vi "tm_getparameterlimits_41.vi"(7 "Reconfigure (F)":bool, 8 "error in (no error)":errorcluster, 10 "Parameter":u32(ring)=4215968 items=["SENSOR MODE"=4212128, "SENSOR MODE LINE BUNDLE HEIGHT"=4212192, "READOUT DIRECTION"=4211904, "BIT PER CHANNEL"=4342976, "EXPOSURE TIME"=2049184, "CONTRAST GAIN"=3163312, "BINNING"=4215968, "TIMING READOUT TIME"=4223904, "INTERNAL FRAME RATE"=4225952, "INTERNAL FRAME INTERVAL"=4225968, "INTERNAL LINE SPEED"=4226000, "IMAGE WIDTH"=4343200, "IMAGE HEIGHT"=4343216, "IMAGE ROWBYTES"=4343232, "IMAGE FRAMEBYTES"=4343248, "IMAGE PIXEL TYPE"=4343296], 11 "Handle in":u32) -> (0 "error out":errorcluster, 2 "Limits":T1, 3 "Handle out":u32)   [LabVIEW 2023]
uses:
  tmcamcon.dll
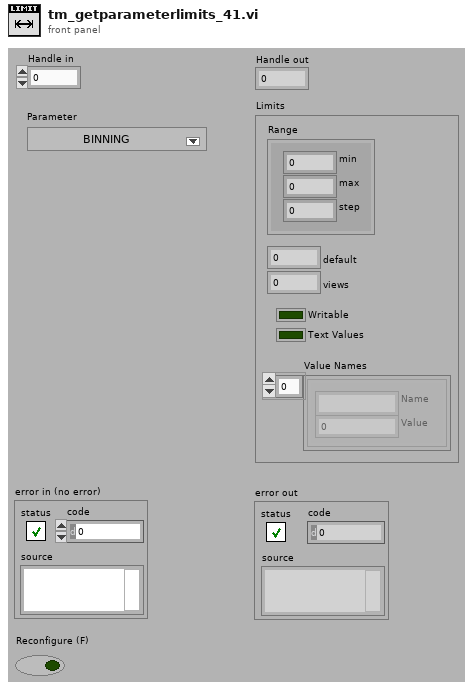
[diagram p1: front panel]
types:
  T1 = cluster{"Range":cluster{"min":dbl, "max":dbl, "step":dbl}, "default":dbl, "views":u32, "Writable":bool, "Text Values":bool, "Value Names":cluster{"Name":string, "Value":dbl}[]}
  T2 = cluster{"Property Name":string, "Property ID":i32}[]
  T3 = cluster{"Property Name":string, "Property ID":i32}
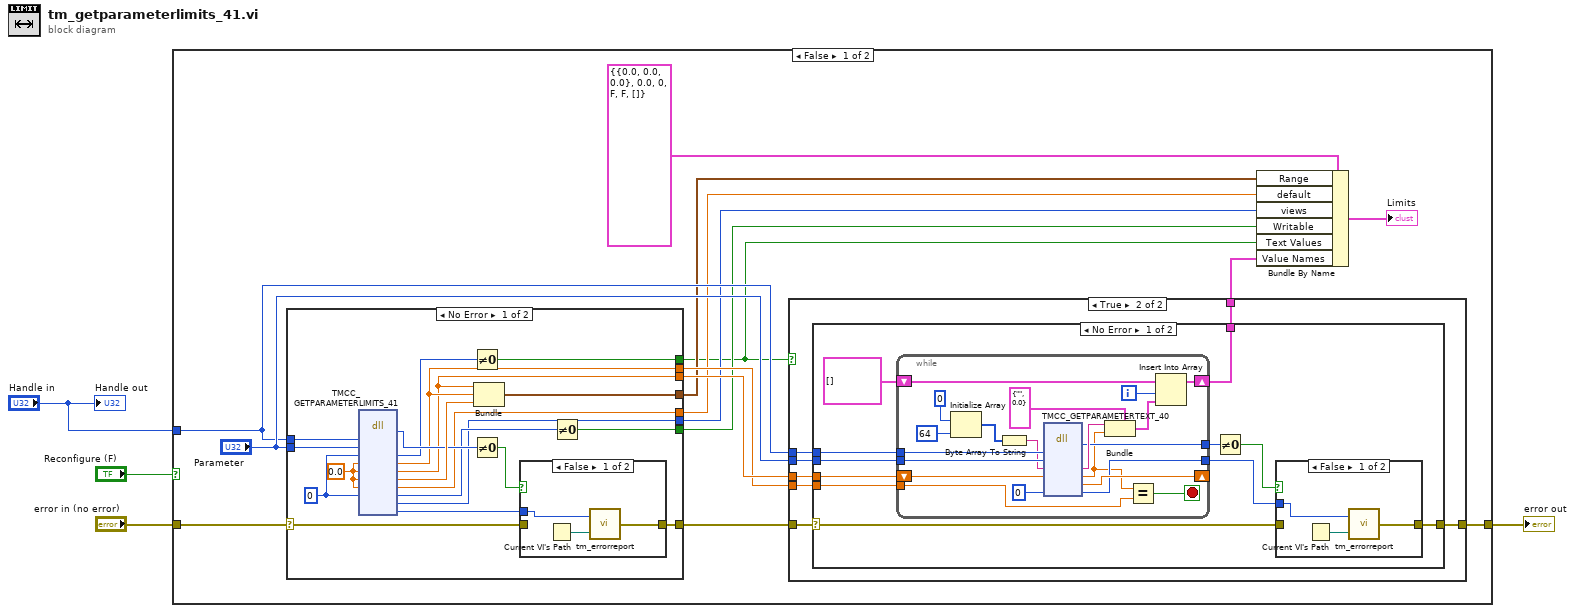
[diagram p0: block diagram]
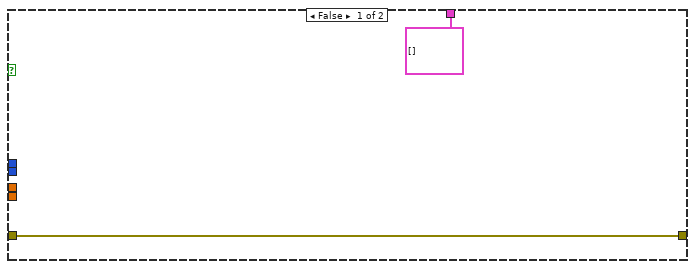
[diagram p2: hidden frame]
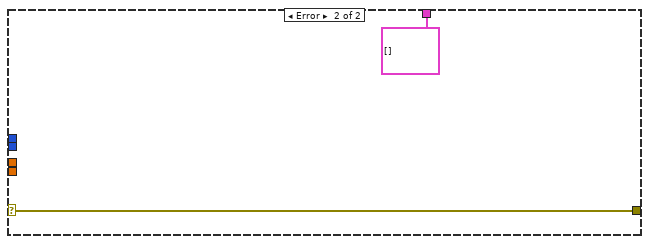
[diagram p4: hidden frame]
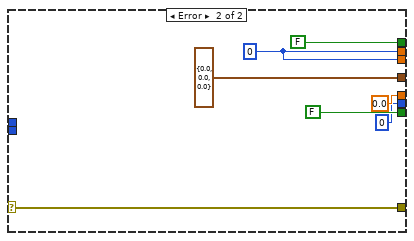
[diagram p6: hidden frame]
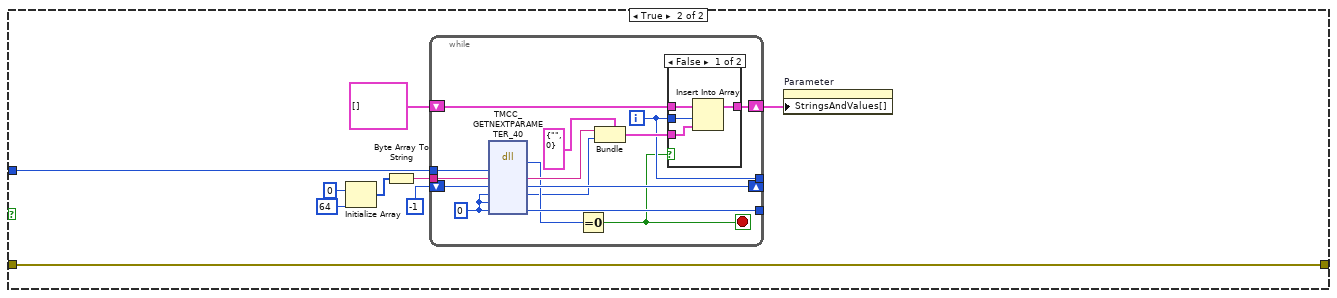
[diagram p7: hidden frame]
diagram:
  n1 = case shown="False" "Reconfigure (F)" {
    tunnel: "error in (no error)" -> [w14 w104]
    tunnel: [w15 w104] -> w3
    tunnel: "Handle in" -> [w13 w96]
    frame False {
      n2 = case shown="No Error" w14 {
        selector: w14 -> [w74 w95]
        tunnel: [w71 w95] -> w16
        tunnel: "Parameter" -> [w84 _]
        tunnel: w13 -> [w79 _]
        tunnel: [w78 w94] -> w17
        tunnel: [w77 w94] -> w18
        tunnel: [w70 FALSE] -> w5
        tunnel: [w69 cluster{"min":dbl, "max":dbl, "step":dbl} {"min"=0.0, "max"=0.0, "step"=0.0}] -> w10
        tunnel: [w68 0.0 ("default")] -> w9
        tunnel: [w67 u32 0 ("views")] -> w8
        tunnel: [w66 FALSE] -> w7
        frame No Error {
          w83 = 0.0
          w75 = u32 0
          n3 = dll-call lib="tmcamcon.dll" fn="TMCC_GETPARAMETERLIMITS_41"("HDCAM"=w79, "propertyid"=w84, "text"=w75, "max"=w83, "min"=w83, "step"=w83, "default"=w83, "writable"=w75) -> ("return type"=w81:u32, "text"=w80:u32, "max"=w78:dbl, "min"=w77:dbl, "step"=w82:dbl, "default"=w68:dbl, "writable"=w76:u32, "views"=w67:u32, "Erval"=w73:i32)  [unwired: 7 in, 2 out]
          n4 = Not Equal To 0?(x=w80) -> (x != 0?=w70:bool)
          n5 = Not Equal To 0?(x=w81) -> (x != 0?=w72:bool)
          n6 = Bundle("min"=w77, "max"=w78, "step"=w82) -> (w69:cluster{"min":dbl, "max":dbl, "step":dbl})  [unwired: 1 in]
          n7 = case shown="False" w72 {
            tunnel: w74 -> [_ w88]
            tunnel: [w86 w88] -> w71
            tunnel: w73 -> [w85 _]
            frame False {
              n8 = Current VI's Path() -> (path=w87:path)
              n9 = call "tm_errorreport.vi"("Source"=w87, "Error"=w85) -> ("error out"=w86:errorcluster)
            }
            frame True {
            }
          }
          n10 = Not Equal To 0?(x=w76) -> (x != 0?=w66:bool)
        }
        frame Error {
          w94 = 0
        }
      }
      n11 = case shown="True" w5 {
        tunnel: w16 -> [w21 w28]
        tunnel: w13 -> [_ w27]
        tunnel: "Parameter" -> [_ w26]
        tunnel: w18 -> [_ w25]
        tunnel: w17 -> [_ w24]
        tunnel: [w21 w23] -> w15
        tunnel: [cluster{"Name":string, "Value":dbl}[] [] ("Value Names") w22] -> w6
        frame False {
        }
        frame True {
          n12 = case shown="No Error" w28 {
            selector: w28 -> [w33 w65]
            tunnel: [w30 w65] -> w23
            tunnel: w27 -> [w37 _]
            tunnel: w26 -> [w36 _]
            tunnel: w25 -> [w35 _]
            tunnel: w24 -> [w34 _]
            tunnel: [w29 cluster{"Name":string, "Value":dbl}[] [] ("Value Names")] -> w22
            frame No Error {
              n13 = while {
                shift-right: [w62] -> w29
                shift-left: cluster{"Name":string, "Value":dbl}[] [] ("Value Names") -> [w63]
                tunnel: [w59] -> w38
                tunnel: w37 -> [w57]
                tunnel: w36 -> [w56]
                shift-right: [w54] -> _
                shift-left: w35 -> [w55]
                tunnel: [w51] -> w32
                tunnel: w34 -> [w50]
                i -> [w58]
                stop <- w48 stop-if-true
                n14 = Initialize Array(u8 0, 64) -> (w45:u8[])
                n15 = Byte Array To String(unsigned byte array=w45) -> (string=w44:string)
                n16 = dll-call lib="tmcamcon.dll" fn="TMCC_GETPARAMETERTEXT_40"("HDCAM"=w57, "propertyid"=w56, "name"=w44, "value"=w55, "Erval"=0) -> ("return type"=w59:u32, "name"=w60:string, "value"=w49:dbl, "nextvalue"=w54:dbl, "Erval"=w51:i32)  [unwired: 6 in, 2 out]
                n17 = Bundle(cluster=cluster{"name":string, "value":dbl} {"name"="", "value"=0.0}, "name"=w60, "value"=w49) -> (w61:cluster{"name":string, "value":dbl})
                n18 = Equal?(x=w49, y=w50) -> (x = y?=w48:bool)
                n19 = Insert Into Array(array=w63, index=w58, new element=w61) -> (w62:cluster{"Name":string, "Value":dbl}[])
              }
              n20 = Not Equal To 0?(x=w38) -> (x != 0?=w31:bool)
              n21 = case shown="False" w31 {
                tunnel: w33 -> [_ w43]
                tunnel: [w41 w43] -> w30
                tunnel: w32 -> [w40 _]
                frame False {
                  n22 = Current VI's Path() -> (path=w42:path)
                  n23 = call "tm_errorreport.vi"("Source"=w42, "Error"=w40) -> ("error out"=w41:errorcluster)
                }
                frame True {
                }
              }
            }
            frame Error {
            }
          }
        }
      }
      n24 = Bundle By Name(cluster=T1 {"Range"={"min"=0.0, "max"=0.0, "step"=0.0}, "default"=0.0, "views"=0, "Writable"=FALSE, "Text Values"=FALSE, "Value Names"=[]} ("Limits"), "Range"=w10, "default"=w9, "views"=w8, "Writable"=w7, "Text Values"=w5, "Value Names"=w6) -> (→"Limits":T1)
    }
    frame True {
      n25 = Initialize Array(u8 0 ("element"), 64 ("dimension size")) -> (w102:u8[])
      n26 = Byte Array To String(unsigned byte array=w102) -> (string=w99:string)
      n27 = while {
        shift-right: [w118] -> w97
        shift-left: T2 [] ("Array") -> [w119]
        tunnel: [w114] -> _
        tunnel: [w112] -> _
        tunnel: w99 -> [w111]
        tunnel: w96 -> [w110]
        shift-right: [w113] -> _
        shift-left: -1 ("func_num") -> [w115]
        i -> [w112]
        stop <- w108 stop-if-true
        w105 = 0 ("option")
        n28 = dll-call lib="tmcamcon.dll" fn="TMCC_GETNEXTPARAMETER_40"("HDCAM"=w110, "name"=w111, "func_num"=w115, "func_id"=w105, "option"=w105, "Erval"=w105) -> ("return type"=w107:u32, "name"=w116:string, "func_num"=w113:i32, "func_id"=w106:i32, "Erval"=w114:i32)  [unwired: 5 in, 2 out]
        n29 = Equal To 0?(x=w107) -> (x = 0?=w108:bool)
        n30 = Bundle(cluster=T3 {"Property Name"="", "Property ID"=0} ("new element/subarray"), "Property Name"=w116, "Property ID"=w106) -> (w117:T3)
        n31 = case shown="False" w108 {
          tunnel: w119 -> [w123 w124]
          tunnel: [w122 w124] -> w118
          tunnel: w112 -> [w121 _]
          tunnel: w117 -> [w120 _]
          frame False {
            n32 = Insert Into Array(array=w123, index=w121, new element=w120) -> (w122:T2)
          }
          frame True {
          }
        }
      }
      n33 = property on="Parameter" class="Ring (strict)"("StringsAndValues[]"=w97) -> ()  [unwired: 2 in, 2 out]
    }
  }
  "error out" <- w3
  "Handle out" <- "Handle in"
